vi "SPI Flash Erase.vi"(5 "TimeOutMs":i32, 6 "EraseCmd":u8, 7 "AddrBytes":u8, 9 "StartAddr":i32, 10 "SPIIndex":i32, 11 "DevHandle":i32) -> (3 "function return":i32)   [LabVIEW 2010, in "usb2spi.lvlib"]
doc: "int WINAPI SPI_FlashErase(int DevHandle,int SPIIndex,int StartAddr,unsigned char AddrBytes,unsigned char EraseCmd,int TimeOutMs);"
uses:
  usb2spi.lvlib
  USB2XXX/trunk/USB2XXX/USB2XXX/vs2019/Release/USB2XXX.dll
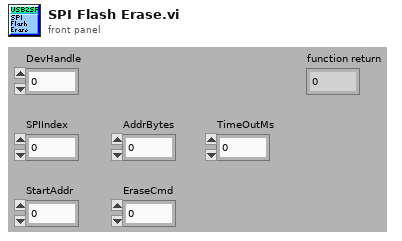
[diagram p1: front panel]
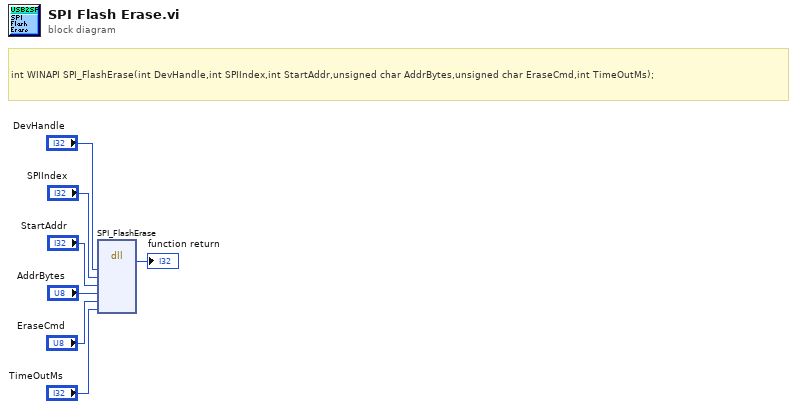
[diagram p0: block diagram]
diagram:
  # "int WINAPI SPI_FlashErase(int DevHandle,int SPIIndex,int StartAddr,unsigned char AddrBytes,unsigned char EraseCmd,int TimeOutMs);"
  n1 = dll-call lib="E:/Projects/USB2XXX/trunk/USB2XXX/USB2XXX/vs2019/Release/USB2XXX.*" fn="SPI_FlashErase"("DevHandle"="DevHandle", "SPIIndex"="SPIIndex", "StartAddr"="StartAddr", "AddrBytes"="AddrBytes", "EraseCmd"="EraseCmd", "TimeOutMs"="TimeOutMs") -> (→"function return":i32)  [unwired: 9 in, 2 out]
